vi "draw_lines.vi"(4 "line_width":i32=8, 6 "line_Color":u32(colorbox)=6618880, 7 "Lanes":cluster{"X":dbl, "Y":dbl}[][](array[cluster]), 8 "error in (no error)":errorcluster, 9 "ROI":cluster{"X":dbl, "Y":dbl}[](array[cluster]), 10 "lines":cluster{"X":dbl, "Y":dbl}[][](array[cluster]), 11 "Image":T1(plugin-control)) -> (0 "error out":errorcluster, 3 "Image out":T1(plugin-control))   [LabVIEW 2021, in "Framework_lib.lvlib"]
uses:
  QMH/Framework_lib.lvlib
  <vilib>/vision/NI_Vision_Development_Module.lvlib
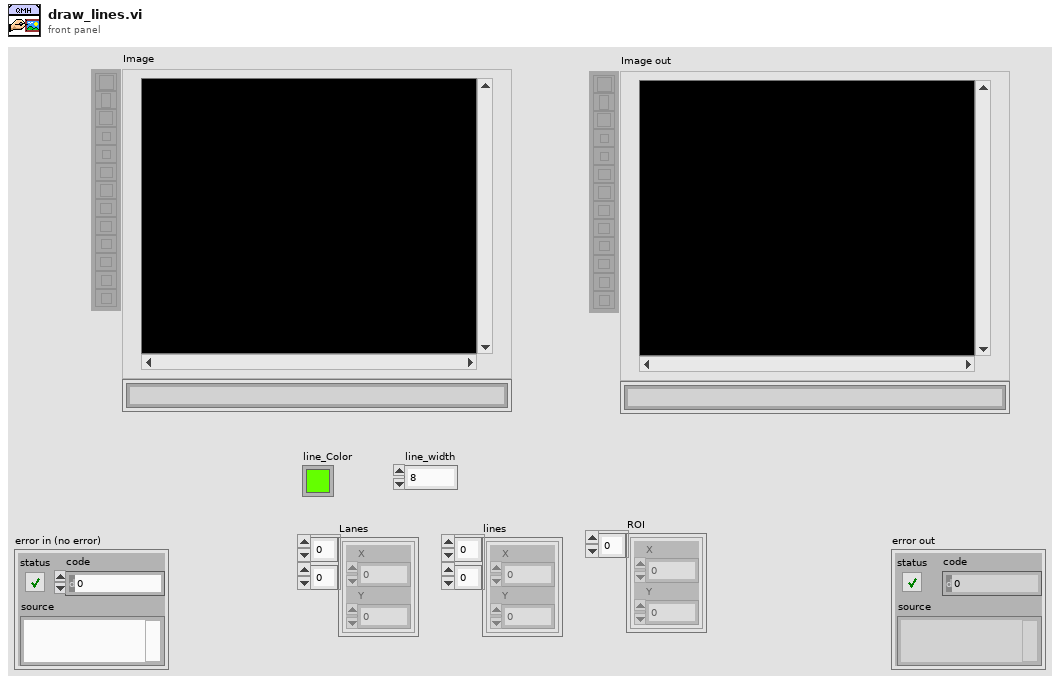
[diagram p1: front panel]
types:
  T1 = typedef "IMAQ Image.ctl" = refnum<image>
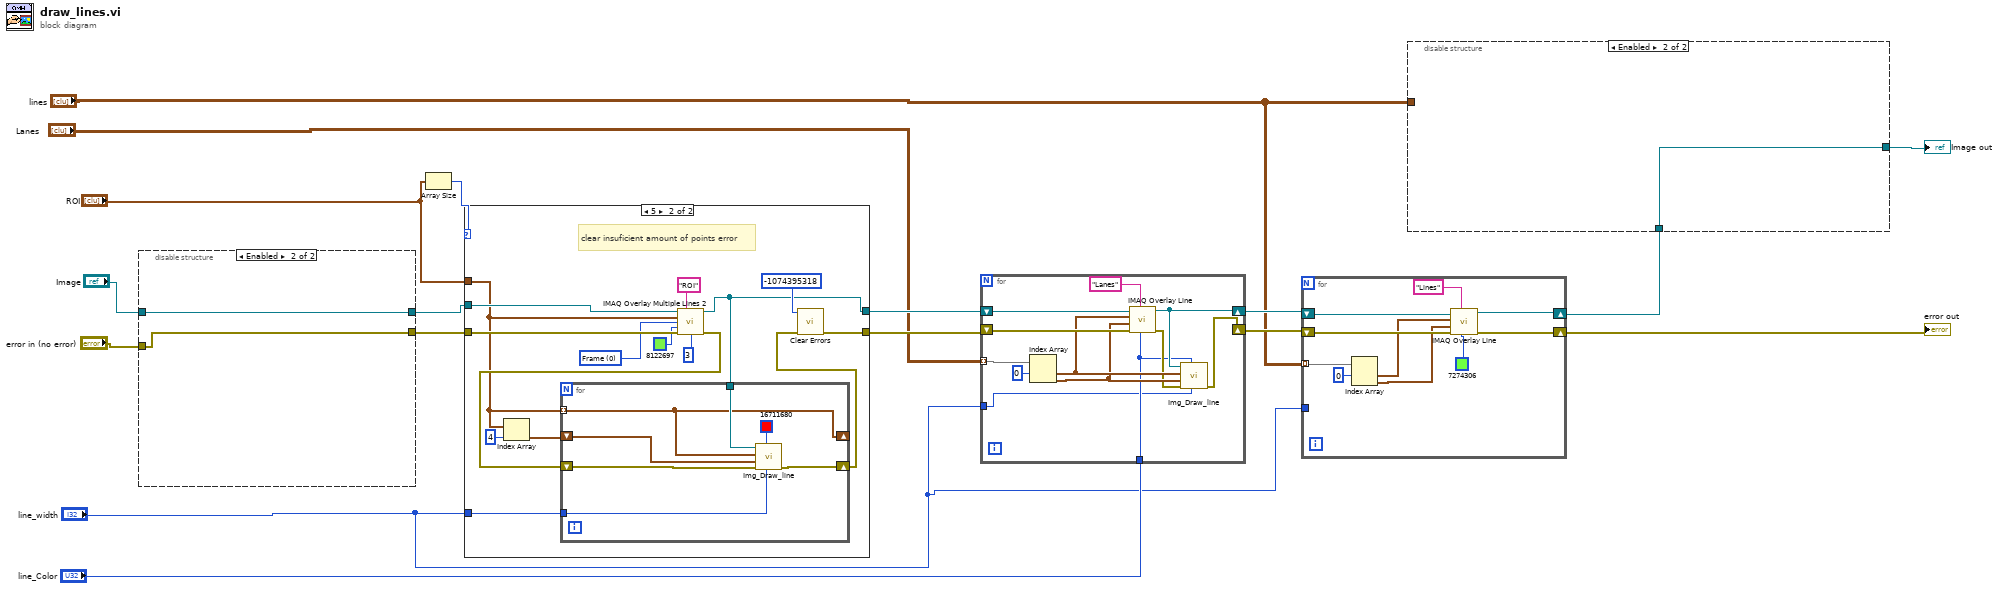
[diagram p0: block diagram]
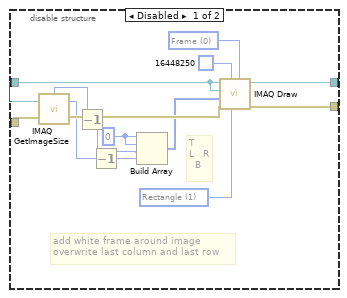
[diagram p2: hidden frame]
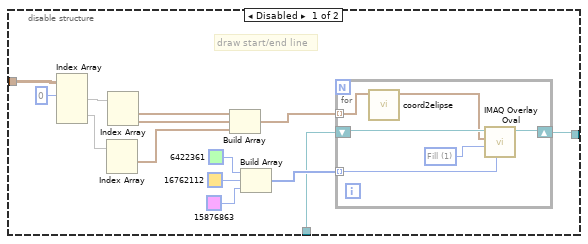
[diagram p3: hidden frame]
diagram:
  n1 = disable-structure shown="Enabled" {
    disable-tunnel: [w31 w33] -> w12
    disable-tunnel: [w30 w32] -> w11
    disable-tunnel: "error in (no error)" -> [w28 w33]
    disable-tunnel: "Image" -> [w26 w32]
    frame Disabled {
      w18 = u16 0 items=["Frame", "Paint", "Invert Frame", "Invert Paint"] ("Draw Mode")
      w23 = 0 ("element")
      w29 = u16 1 items=["Line", "Rectangle", "Oval"] ("Shape to draw")
      # "add white frame around image\noverwrite last column and last row"
      # "T\nL   R\n  B"
      n2 = call "IMAQ GetImageSize"("Image"=w26, "error in (no error)"=w28) -> ("Y Resolution"=w21:i32, "X Resolution"=w22:i32, "error out"=w27:errorcluster)  [unwired: 2 in]
      n3 = Decrement(x=w22) -> (x-1=w19:i32)
      n4 = Decrement(x=w21) -> (x-1=w20:i32)
      n5 = Build Array(w23, w23, w19, w20) -> (w24:i32[])
      n6 = call "IMAQ Draw"("Draw Mode"=w18, "Shape to draw"=w29, "Pixel Color"=u32 16448250 ("Color"), "error in (no error)"=w27, "Coordinates"=w24, "Image Dst"=w26, "Image Src"=w26) -> ("error out"=w31:errorcluster, "Image Dst Out"=w30:T1)  [unwired: 3 in]
    }
    frame Enabled {
    }
  }
  n7 = Array Size(array="ROI") -> (size(s)=w15:i32)
  n8 = case shown="5" w15 {
    tunnel: [w34 w50] -> w17
    tunnel: [w35 w40] -> w16
    tunnel: w11 -> [w35 w49]
    tunnel: w12 -> [w34 w48]
    tunnel: "ROI" -> [_ w38]
    tunnel: "line_width" -> [_ w36]
    frame 0, Default {
    }
    frame 5 {
      w45 = u32 0 items=["Frame", "Fill"] ("Drawing Mode (Frame)")
      # "clear insuficient amount of points error"
      n9 = Index Array(array=w38, index=4) -> (element=w39:cluster{"X":dbl, "Y":dbl})
      n10 = call "IMAQ Overlay Multiple Lines 2"("Image"=w49, "Group"="ROI", "Line End Points"=w38, "Drawing Mode (Frame)"=w45, "Color"=u32 8122697, "error in (no error)"=w48, "Width"=u32 3) -> ("Image Out"=w40:T1, "error out"=w42:errorcluster)  [unwired: 7 in]
      n11 = for {
        tunnel: w40 -> [w55]
        shift-right: [w56] -> w41
        shift-left: w42 -> [w57]
        shift-right: [w53] -> _
        shift-left: w39 -> [w52]
        tunnel: w38 -> [w53] mode=indexing
        tunnel: w36 -> [w51]
        n12 = call "Img_Draw_line.vi"("line_width"=w51, "Color"=u32 16711680, "error in (no error)"=w57, "Point Coordinates 2"=w52, "Point Coordinates 1"=w53, "Img In"=w55) -> ("error out"=w56:errorcluster)  [unwired: 4 in, 1 out]
      }
      n13 = call <vilib>:"Clear Errors.vi"("error in (no error)"=w41, "specific error code to clear (0: all)"=-1074395318) -> ("error out"=w50:errorcluster)  [unwired: 4 in, 1 out]
    }
  }
  n14 = for {
    tunnel: "Lanes" -> [w67] mode=indexing
    shift-right: [w64] -> w6
    shift-left: w16 -> [w69]
    shift-right: [w60] -> w5
    shift-left: w17 -> [w68]
    tunnel: "line_Color" -> [w59]
    tunnel: "line_width" -> [w58]
    n15 = Index Array(array=w67, index #1=0 ("index")) -> (element #1=w63:cluster{"X":dbl, "Y":dbl}, element #2=w62:cluster{"X":dbl, "Y":dbl})  [unwired: 1 in]
    n16 = call "IMAQ Overlay Line"("Color"=w59, "Group"="Lanes", "error in (no error)"=w68, "End Point"=w62, "Start Point"=w63, "Image"=w69) -> ("error out"=w61:errorcluster, "Image Out"=w64:T1)  [unwired: 4 in]
    n17 = call "Img_Draw_line.vi"("line_width"=w58, "Color"=w59, "error in (no error)"=w61, "Point Coordinates 2"=w62, "Point Coordinates 1"=w63, "Img In"=w64) -> ("error out"=w60:errorcluster)  [unwired: 4 in, 1 out]
  }
  n18 = for {
    shift-right: [w75] -> w1
    shift-left: w6 -> [w79]
    shift-right: [w71] -> w2
    shift-left: w5 -> [w78]
    tunnel: "line_width" -> [_]
    tunnel: "lines" -> [w72] mode=indexing
    n19 = Index Array(array=w72, index #1=0 ("index")) -> (element #1=w74:cluster{"X":dbl, "Y":dbl}, element #2=w73:cluster{"X":dbl, "Y":dbl})  [unwired: 1 in]
    n20 = call "IMAQ Overlay Line"("Color"=u32 7274306, "Group"="Lines", "error in (no error)"=w78, "End Point"=w73, "Start Point"=w74, "Image"=w79) -> ("error out"=w71:errorcluster, "Image Out"=w75:T1)  [unwired: 4 in]
  }
  "error out" <- w2
  n21 = disable-structure shown="Enabled" {
    disable-tunnel: w1 -> [w84 w100]
    disable-tunnel: "lines" -> [w81 _]
    disable-tunnel: [w80 w100] -> w13
    frame Disabled {
      # "draw start/end line"
      n22 = Index Array(array=w81, index (row) #1=0 ("index")) -> (element #1=w83:cluster{"X":dbl, "Y":dbl}[], element #2=w91:cluster{"X":dbl, "Y":dbl}[])  [unwired: 3 in]
      n23 = Index Array(array=w91) -> (element #1=w92:cluster{"X":dbl, "Y":dbl})  [unwired: 2 in, 1 out]
      n24 = Index Array(array=w83) -> (element #1=w85:cluster{"X":dbl, "Y":dbl}, element #2=w87:cluster{"X":dbl, "Y":dbl})  [unwired: 2 in]
      n25 = Build Array(w85, w87, w92) -> (w86:cluster{"X":dbl, "Y":dbl}[])
      n26 = Build Array(u32 6422361 ("Color"), u32 16762112 ("Color"), u32 15876863 ("Color")) -> (w89:u32[])
      n27 = for {
        tunnel: w86 -> [w96] mode=indexing
        shift-right: [w98] -> w80
        shift-left: w84 -> [w99]
        tunnel: w89 -> [w94] mode=indexing
        w97 = u32 1 items=["Frame", "Fill"] ("Drawing Mode (Frame)")
        n28 = call "coord2elipse.vi"("Point Coordinates"=w96) -> ("Cluster"=w95:cluster{dbl, dbl, dbl, dbl})  [unwired: 10 in]
        n29 = call "IMAQ Overlay Oval"("Color"=w94, "Drawing Mode (Frame)"=w97, "Bounding Rectangle"=w95, "Image"=w99) -> ("Image Out"=w98:T1)  [unwired: 6 in, 1 out]
      }
    }
    frame Enabled {
    }
  }
  "Image out" <- w13
